vi "manip_status_test.vi"() -> ()   [LabVIEW 2014]
doc: "The UDP protocol differs from TCP in that there is no error-checking with the packets of information that are sent, and thus no guarantee whatsoever that an intended recipient will actually receive a given piece of data.\n\nUDP does offer the ability to \"broadcast\" data across a network--simply specify an IP Address of all ones (255.255.255.255) to attempt to broadcast information network-wide. Keep in mind that routers and other network hardware will generally refuse to forward the broadcast beyond certain points, so the extent of the broadcast will in practice be limited."
panel:
  out "length":i32
  out "Rx packets":i32
  in  "receiver port":u16=61559
  out "Array":u32[](array[numeric])
  in  "Stop":bool
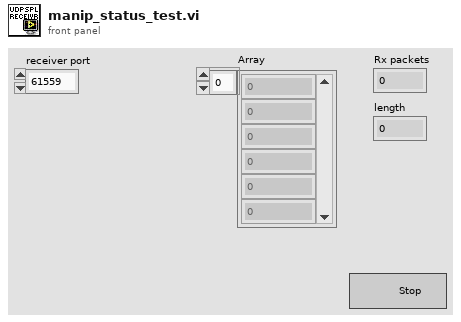
[diagram p1: front panel]
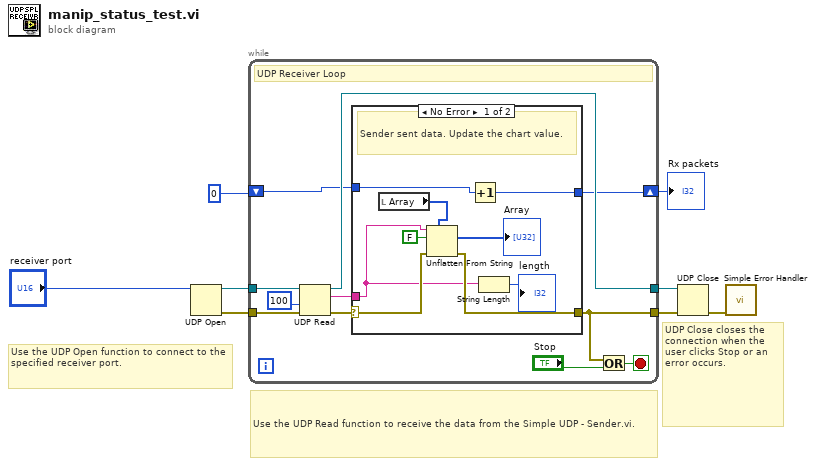
[diagram p0: block diagram]
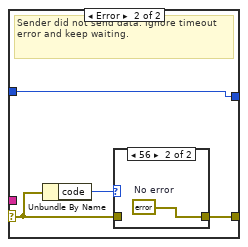
[diagram p2: hidden frame]
diagram:
  # "UDP Close closes the connection when the user clicks Stop or an error occurs."
  # "Use the UDP Open function to connect to the specified receiver port."
  # "Use the UDP Read function to receive the data from the Simple UDP - Sender.vi."
  n1 = UDP Open(11:"receiver port") -> (port=w4:refnum<k16>, 0:w5:errorcluster)  [unwired: 4 in, 1 out]
  n2 = while {
    tunnel: w4 -> [w19]
    tunnel: [w11] -> w8
    tunnel: w5 -> [w16]
    tunnel: [w12] -> w6
    shift-right: [w9] -> w1
    shift-left: 0 -> [w10]
    stop <- w17 stop-if-true
    # "UDP Receiver Loop"
    n3 = UDP Read(connection ID=w19, timeout ms (25000)=100, 8:w16) -> (data out=w14:string, error out=w13:errorcluster, 3:w11:refnum<k16>)  [unwired: 3 out]
    n4 = case shown="No Error" w13 {
      selector: w13 -> [w25 w31]
      tunnel: w14 -> [w21 _]
      tunnel: [w24 w30] -> w12
      tunnel: w10 -> [w23 w29]
      tunnel: [w22 w29] -> w9
      frame No Error {
        # "Sender sent data. Update the chart value."
        n5 = local read "Array"() -> (w26:u32[])
        n6 = Unflatten From String(type=w26, binary string=w21, data includes array or string size? (T)=FALSE, error in (no error)=w25) -> (value=→"Array":u32[], error out=w24:errorcluster)  [unwired: 1 in, 1 out]
        n7 = Increment(x=w23) -> (x+1=w22:i32)
        n8 = String Length(string=w21) -> (length=→"length":i32)
      }
      frame Error {
        # "Sender did not send data. Ignore timeout error and keep waiting."
        n9 = Unbundle By Name(w31) -> ("code"=w32:i32)
        n10 = case shown="56" w32 {
          tunnel: w31 -> [w33 _]
          tunnel: [w33 w34] -> w30
          frame Default {
          }
          frame 56 {
            w34 = errorcluster {"status"=FALSE, "code"=0, "source"=""}  # No error
          }
        }
      }
    }
    n11 = Or(x=w12, y="Stop") -> (x .or. y?=w17:bool)
  }
  "Rx packets" <- w1
  n12 = UDP Close(connection ID=w8, 8:w6) -> (error out=w7:errorcluster)  [unwired: 1 out]
  n13 = call <vilib>:"Simple Error Handler.vi"("error in (no error)"=w7) -> ()  [unwired: 1 in, 8 out]
